vi "FB_Enable.vi"(8 "error in":errorcluster, 11 "Python":T1) -> (0 "error out":errorcluster, 2 "Reply":string, 3 "Python":T1)   [LabVIEW 2022 SP3]
uses:
  PythonCtrl.ctl
  Processors.ctl
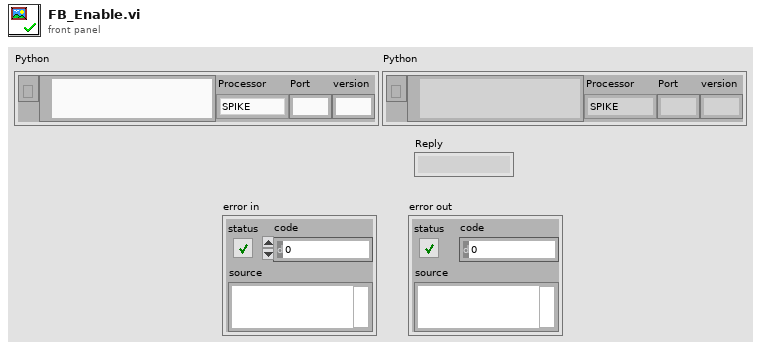
[diagram p1: front panel]
types:
  T1 = typedef "PythonCtrl.ctl" = cluster{"session":refnum<k35>, "PyPath":path, "Processor":T2, "Port":string, "version":string}
  T2 = typedef "Processors.ctl" = enum16{"SPIKE", "Pi", "Pi_ssh", "OpenMV", "Dunio"}
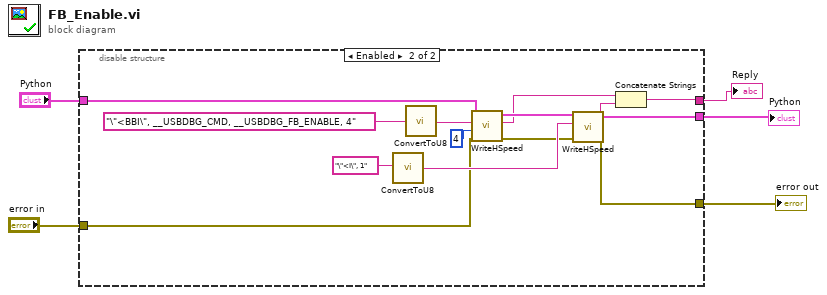
[diagram p0: block diagram]
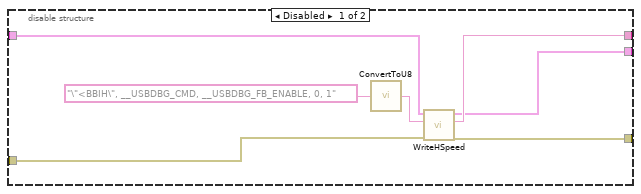
[diagram p2: hidden frame]
diagram:
  n1 = disable-structure shown="Enabled" {
    disable-tunnel: "Python" -> [w12 w22]
    disable-tunnel: "error in" -> [w11 w15]
    disable-tunnel: [w10 w18] -> w3
    disable-tunnel: [w7 w21] -> w2
    disable-tunnel: [w6 w13] -> w1
    frame Disabled {
      n2 = call "ConvertToU8.vi"("struct"="\"<BBIH\", __USBDBG_CMD, __USBDBG_FB_ENABLE, 0, 1" ("write buffer")) -> ("Binary"=w8:string)
      n3 = call "WriteHSpeed.vi"("error in"=w11, "write buffer"=w8, "Python"=w12) -> ("error out"=w6:errorcluster, "read buffer"=w10:string, "Python"=w7:T1)  [unwired: 6 in]
    }
    frame Enabled {
      n4 = call "ConvertToU8.vi"("struct"="\"<I\", 1" ("write buffer")) -> ("Binary"=w16:string)
      n5 = call "ConvertToU8.vi"("struct"="\"<BBI\", __USBDBG_CMD, __USBDBG_FB_ENABLE, 4" ("write buffer")) -> ("Binary"=w25:string)
      n6 = call "WriteHSpeed.vi"("error in"=w15, "Reply length"=4, "write buffer"=w25, "Python"=w22) -> ("error out"=w14:errorcluster, "read buffer"=w20:string, "Python"=w23:T1)  [unwired: 5 in]
      n7 = call "WriteHSpeed.vi"("error in"=w14, "write buffer"=w16, "Python"=w23) -> ("error out"=w13:errorcluster, "read buffer"=w19:string, "Python"=w21:T1)  [unwired: 6 in]
      n8 = Concatenate Strings(w20, w19) -> (w18:string)
    }
  }
  "error out" <- w1
  "Python" <- w2
  "Reply" <- w3
